vi "TEST_TCP_DATA_Subscriber.vi"() -> (0 "error out":errorcluster={"status"=TRUE, "code"=66, "source"="TCP Read in test_DATA_TCP_client.vi"}, 8 "error in":errorcluster)   [LabVIEW 2009]
panel:
  out "NaN/Path/Refnum?":bool
  out "error out 2":errorcluster
  in  "millisecond multiple":u32=25
  out "data string":string
  in  "stop":bool
  out "after substring 2":string
  out "after substring":string
  out "array":dbl[](graph)
  out "time string":string="4:31 PM"
  out "data out":string
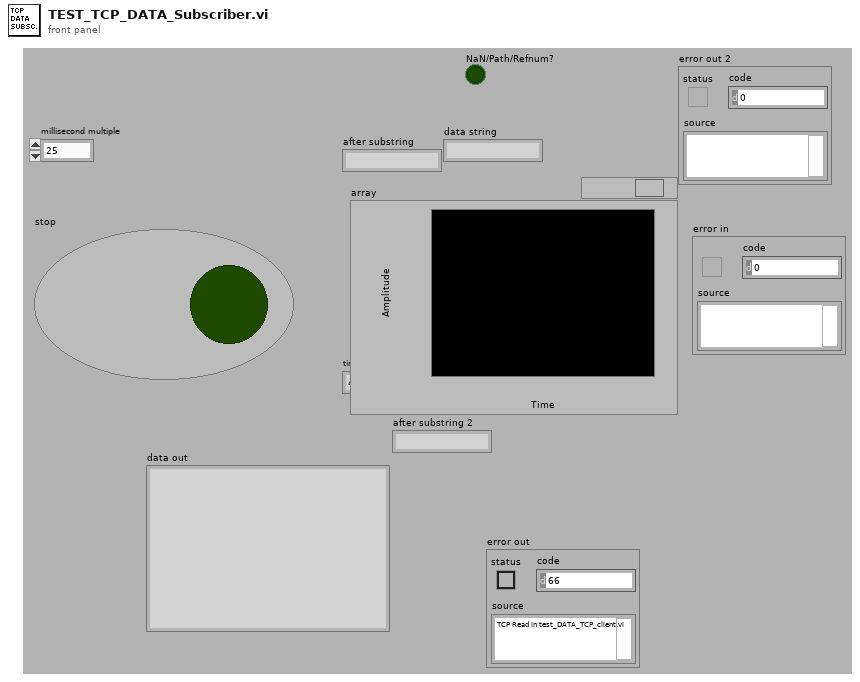
[diagram p1: front panel]
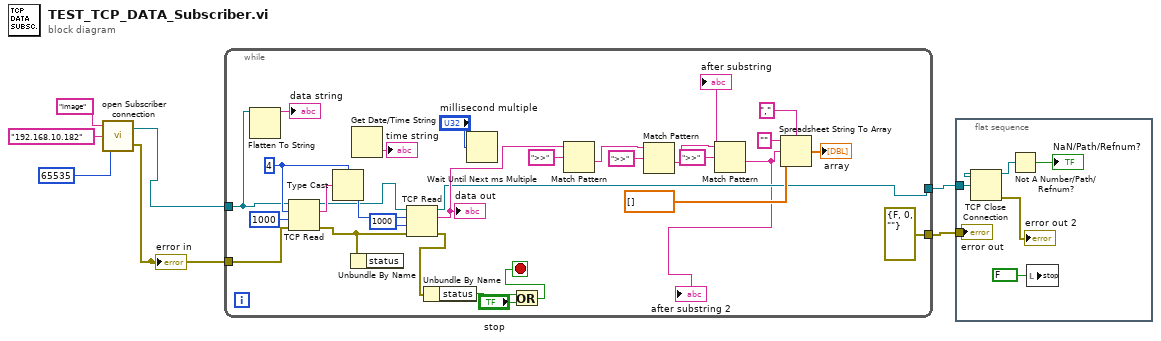
[diagram p0: block diagram]
diagram:
  n1 = call "open Subscriber connection.vi"("Port"=u16 65535, "Machine"="192.168.10.182", "Subscriber list"="image") -> ("error out"=w1:errorcluster, "connection ID"=w3:refnum<k5>)
  "error in" <- w1
  n2 = while {
    tunnel: w1 -> [w30]
    tunnel: w3 -> [w9]
    tunnel: [errorcluster {"status"=FALSE, "code"=0, "source"=""} ("error out")] -> w7
    tunnel: [w16] -> w2
    stop <- w11 stop-if-true
    w35 = 4
    n3 = Flatten To String(anything=w9) -> (data string=→"data string":string)  [unwired: 3 in, 2 out]
    n4 = TCP Read(connection ID=w9, bytes to read=w35, error in (no error)=w30, 9:1000 ("timeout ms (25000)")) -> (connection ID out=w32:refnum<k5>, data out=w34:string, error out=w29:errorcluster)  [unwired: 1 in]
    n5 = Type Cast(type=w35, x=w34) -> (*(type *) &x=w33:i32)
    n6 = Unbundle By Name(w29) -> ()  [unwired: 1 out]
    n7 = Get Date/Time String() -> (time string=→"time string":string)  [unwired: 3 in, 1 out]
    n8 = TCP Read(connection ID=w32, bytes to read=w33, error in (no error)=w29, 9:1000) -> (connection ID out=w16:refnum<k5>, data out=w26:string, error out=w14:errorcluster)  [unwired: 1 out]
    "data out" <- w26
    n9 = Unbundle By Name(w14) -> ("status"=w12:bool)
    n10 = Wait Until Next ms Multiple(millisecond multiple="millisecond multiple") -> ()  [unwired: 1 out]
    n11 = Or(x=w12, y="stop") -> (x .or. y?=w11:bool)
    n12 = Match Pattern(string=w26, regular expression=">>") -> (after substring=w23:string)  [unwired: 1 in, 3 out]
    n13 = Match Pattern(string=w23, regular expression=">>") -> (after substring=w21:string)  [unwired: 1 in, 3 out]
    n14 = Match Pattern(string=w21, regular expression=">>") -> (after substring=w15:string)  [unwired: 1 in, 3 out]
    "after substring" <- w15
    "after substring 2" <- w15
    n15 = Spreadsheet String To Array(delimiter (Tab)=",", format string="", spreadsheet string=w15, array type (2D Dbl)=dbl[] []) -> (array=→"array":dbl[])
  }
  n16 = flat-sequence {
    tunnel: w7 -> [w42]
    tunnel: w2 -> [w41]
    frame #0 {
      n17 = TCP Close Connection(connection ID=w41) -> (connection ID out=w38:refnum<k5>, error out=→"error out 2":errorcluster)  [unwired: 2 in]
      n18 = Not A Number/Path/Refnum?(number/path/refnum=w38) -> (NaN/Path/Refnum?=→"NaN/Path/Refnum?":bool)
      n19 = local write "stop"(FALSE ("stop")) -> ()
      "error out" <- w42
    }
  }
